vi "Bloomy BS120x Configuration Example.vi"() -> ()   [LabVIEW 2021]
uses:
  src/TypeDefs/UnitType.ctl
  src/TypeDefs/CAN Settings.ctl
  src/TypeDefs/Ethernet Settings.ctl
  src/TypeDefs/Protocol.ctl
  src/Public/New BS120x Device/New BS120x Ethernet Device.vi
  src/BS120x.lvclass
  src/BS120x Driver.lvlib
panel:
  out "reset status":string
  out "Cell Inhibit Enable":bool
  in  "Cell Inhibit Enable":bool
  out "error out":errorcluster
  in  "Reset Unit":bool
  in  "Update IP":bool
  in  "New IP Address":string="192.168.1.100"
  in  "Update Config":bool
  in  "New Protocol (Legacy)":T1 caption="Protocol (Legacy)"
  in  "New Ethernet Settings":T2 caption="Ethernet Settings"
  in  "New CAN Settings":T3 caption="CAN Settings"
  out "Calibration Date":string
  out "SerialNumber":string
  out "Firmware":string
  out "Protocol (Legacy)":T1
  out "Ethernet Settings":T2
  out "CAN Settings":T3
  in  "Retrieve Config":bool
  in  "Box IP address":string="192.168.1.101"
  in  "TCP port":u16=12345
  in  "UDP port":u16=54321
  in  "Unit Type":T4=enum."BS1201"
  in  "stop":bool
  # "Initialization & Configuration"
  # "New Configuration"
  # "Ethernet Only"
  # "Changes do not take effect until unit is reset"
  # "Current Configuration"
  # "Automatically resets unit"
  # "(c) 2024 Bloomy Controls, Inc. All rights reserved."
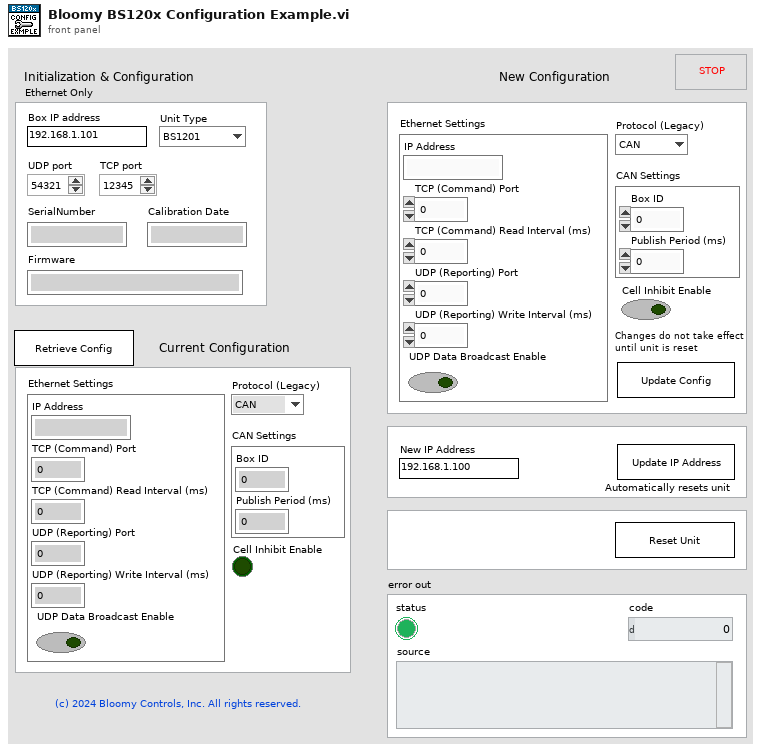
[diagram p1: front panel]
types:
  T1 = typedef "BS120x Driver.lvlib/BS120x.lvclass/Protocol.ctl" = enum16{"CAN", "Ethernet"}
  T2 = typedef "BS120x Driver.lvlib/BS120x.lvclass/Ethernet Settings.ctl" = cluster{"IP Address":string, "TCP (Command) Port":u16, "TCP (Command) Read Interval (ms)":u32, "UDP (Reporting) Port":u16, "UDP (Reporting) Write Interval (ms)":u32, "UDP Data Broadcast Enable":bool}
  T3 = typedef "BS120x Driver.lvlib/BS120x.lvclass/CAN Settings.ctl" = cluster{"Box ID":i32, "Publish Period (ms)":i32}
  T4 = typedef "BS120x Driver.lvlib/BS120x.lvclass/UnitType.ctl" = enum16{"BS1200", "BS1201"}
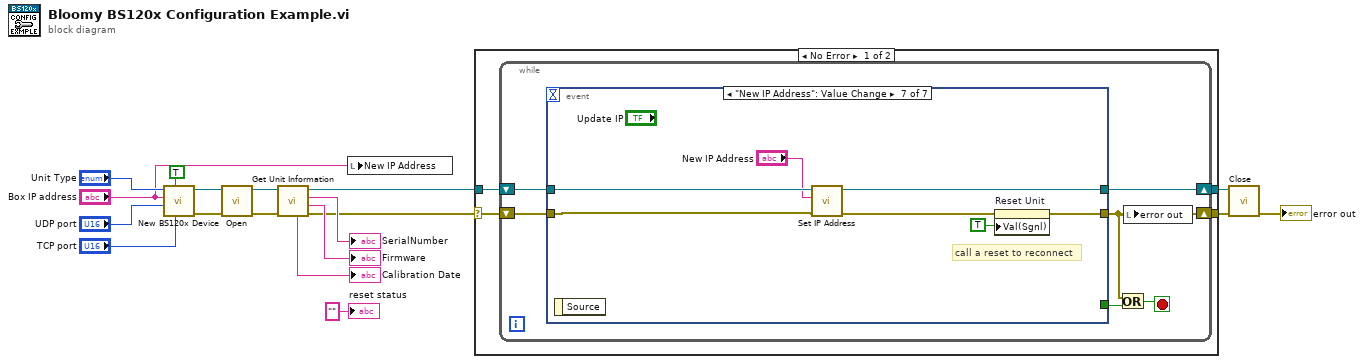
[diagram p0: block diagram]
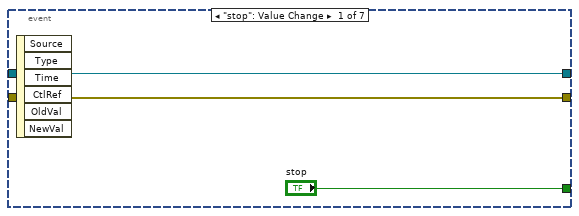
[diagram p2: hidden frame]
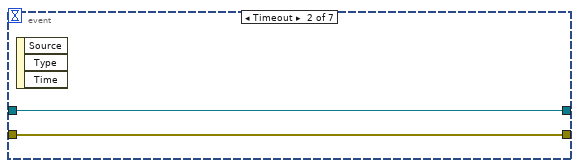
[diagram p3: hidden frame]
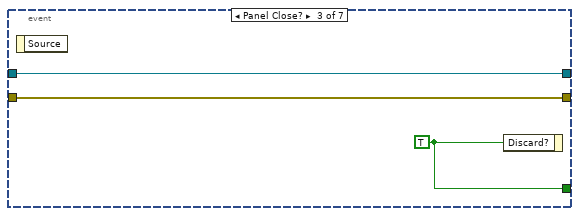
[diagram p4: hidden frame]
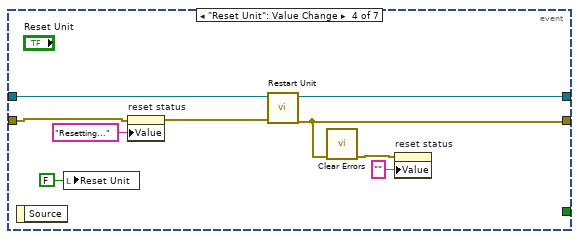
[diagram p5: hidden frame]
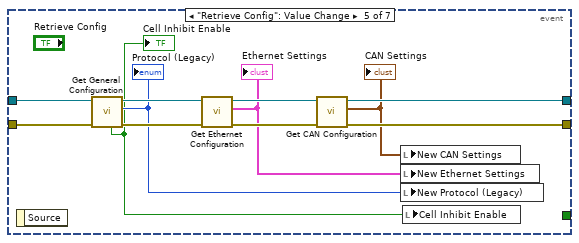
[diagram p6: hidden frame]
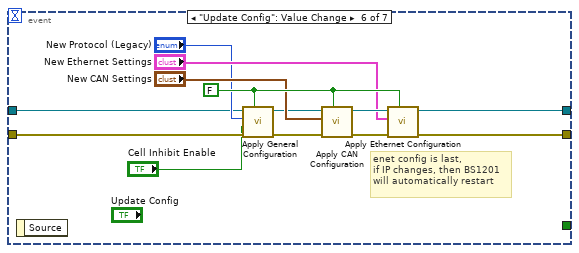
[diagram p7: hidden frame]
diagram:
  n1 = call-poly "New BS120x Device.vi"("TCP port"="TCP port", "Connect for Config Only? (F)"=TRUE, "UDP port"="UDP port", "Box IP address"="Box IP address", "Unit Type"="Unit Type") -> ("error out"=w8:errorcluster, "BS120x Out"=w9:refnum<class "BS120x.lvclass">)  [unwired: 5 in]
  n2 = call-dynamic "Open.vi"("error in (no error)"=w8, "BS120x in"=w9) -> ("error out"=w7:errorcluster, "BS120x out"=w6:refnum<class "BS120x.lvclass">)  [unwired: 8 in]
  n3 = call-dynamic "Get Unit Information.vi"("error in (no error)"=w7, "BS120x in"=w6) -> ("error out"=w2:errorcluster, "Firmware"=→"Firmware":string, "SerialNumber"=→"SerialNumber":string, "BS120x out"=w13:refnum<class "BS120x.lvclass">, "Calibration Date"=→"Calibration Date":string)  [unwired: 5 in]
  n4 = local write "New IP Address"("Box IP address") -> ()
  n5 = case shown="No Error" w2 {
    selector: w2 -> [w19 w78]
    tunnel: [w22 w78] -> w18
    tunnel: [w21 w79] -> w17
    tunnel: w13 -> [w20 w79]
    frame No Error {
      n6 = while {
        shift-right: [w23] -> w22
        shift-left: w19 -> [w26]
        shift-right: [w28] -> w21
        shift-left: w20 -> [w27]
        stop <- w25 stop-if-true
        n7 = event shown="[6] \"New IP Address\": Value Change" {
          selector: _ -> [_ _ _ _ _ _ _]
          dyn-events: _ -> [_ _ _ _ _ _ _]
          timeout: _ -> [_ _ _ _ _ _ _]
          tunnel: [w31 w33 w36 w45 w51 w64 w76] -> w28
          tunnel: w27 -> [w31 w33 w36 w44 w57 w60 w77]
          tunnel: [w30 w32 w34 w40 w50 w63 w72] -> w23
          tunnel: w26 -> [w30 w32 w34 w42 w56 w59 w74]
          tunnel: ["stop" _ w35 _ _ _ _] -> w24
          event "stop": Value Change {
            n8 = event-data() -> ()  [unwired: 1 in, 6 out]
          }
          event Timeout {
            n9 = event-data() -> ()  [unwired: 1 in, 3 out]
          }
          event Panel Close? {
            w35 = TRUE ("Discard?")
            n10 = event-data() -> ()  [unwired: 1 in, 1 out]
            n11 = event-data("Discard?"=w35) -> ()  [unwired: 1 in, 1 out]
          }
          event "Reset Unit": Value Change {
            n12 = event-data() -> ()  [unwired: 1 in, 1 out]
            n13 = local write "Reset Unit"(FALSE ("Reset Unit")) -> ()
            n14 = property on="reset status" class="Str"(error in=w42, "Value"="Resetting..." ("reset status")) -> (error out=w41:errorcluster)  [unwired: 1 in, 1 out]
            n15 = call-dynamic "Restart Unit.vi"("error in (no error)"=w41, "BS120x in"=w44) -> ("error out"=w40:errorcluster, "BS120x out"=w45:refnum<class "BS120x.lvclass">)  [unwired: 8 in]
            n16 = call <vilib>:"Clear Errors.vi"("error in (no error)"=w40) -> ("error out"=w38:errorcluster)  [unwired: 5 in, 1 out]
            n17 = property on="reset status" class="Str"(error in=w38, "Value"="" ("reset status")) -> ()  [unwired: 1 in, 2 out]
          }
          event "Retrieve Config": Value Change {
            n18 = event-data() -> ()  [unwired: 1 in, 1 out]
            n19 = call-dynamic "Get General Configuration.vi"("error in (no error)"=w56, "BS120x in"=w57) -> ("error out"=w54:errorcluster, "Protocol"=w47:T1, "BS120x out"=w55:refnum<class "BS120x.lvclass">, "Cell Inhibit Enable"=w46:bool)  [unwired: 5 in, 1 out]
            "Protocol (Legacy)" <- w47
            "Cell Inhibit Enable" <- w46
            n20 = call-dynamic "Get Ethernet Configuration.vi"("error in (no error)"=w54, "BS120x in"=w55) -> ("error out"=w52:errorcluster, "Ethernet Settings"=w48:T2, "BS120x out"=w53:refnum<class "BS120x.lvclass">)  [unwired: 6 in, 1 out]
            "Ethernet Settings" <- w48
            n21 = call-dynamic "Get CAN Configuration.vi"("error in (no error)"=w52, "BS120x in"=w53) -> ("error out"=w50:errorcluster, "CAN Settings"=w49:T3, "BS120x out"=w51:refnum<class "BS120x.lvclass">)  [unwired: 6 in, 1 out]
            "CAN Settings" <- w49
            n22 = local write "New CAN Settings"(w49) -> ()
            n23 = local write "New Ethernet Settings"(w48) -> ()
            n24 = local write "New Protocol (Legacy)"(w47) -> ()
            n25 = local write "Cell Inhibit Enable"(w46) -> ()
          }
          event "Update Config": Value Change {
            w68 = FALSE ("Restart (T)")
            # "enet config is last,\nif IP changes, then BS1201\nwill automatically restart"
            n26 = event-data() -> ()  [unwired: 1 in, 1 out]
            n27 = call-dynamic "Apply General Configuration.vi"("Restart (T)"=w68, "error in (no error)"=w59, "Cell Inhibit Enable"="Cell Inhibit Enable", "Protocol (Legacy)"="New Protocol (Legacy)", "BS120x in"=w60) -> ("error out"=w61:errorcluster, "BS120x out"=w62:refnum<class "BS120x.lvclass">)  [unwired: 5 in]
            n28 = call-dynamic "Apply CAN Configuration.vi"("Restart (T)"=w68, "error in (no error)"=w61, "CAN Settings"="New CAN Settings", "BS120x in"=w62) -> ("error out"=w69:errorcluster, "BS120x out"=w70:refnum<class "BS120x.lvclass">)  [unwired: 6 in]
            n29 = call-dynamic "Apply Ethernet Configuration.vi"("Restart (T)"=w68, "error in (no error)"=w69, "Ethernet Settings"="New Ethernet Settings", "BS120x in"=w70) -> ("error out"=w63:errorcluster, "BS120x out"=w64:refnum<class "BS120x.lvclass">)  [unwired: 6 in]
          }
          event "New IP Address": Value Change {
            # "call a reset to reconnect"
            n30 = event-data() -> ()  [unwired: 1 in, 1 out]
            n31 = call-dynamic "Set IP Address.vi"("error in (no error)"=w74, "IP Address"="New IP Address", "BS120x in"=w77) -> ("error out"=w73:errorcluster, "BS120x out"=w76:refnum<class "BS120x.lvclass">)  [unwired: 7 in]
            n32 = property on="Reset Unit" class="Bool (strict)"(error in=w73, "Val(Sgnl)"=TRUE ("Value (Signaling)")) -> (error out=w72:errorcluster)  [unwired: 1 in, 1 out]
          }
        }
        n33 = Or(x=w23, y=w24) -> (x .or. y?=w25:bool)
        n34 = local write "error out"(w23) -> ()
      }
    }
    frame Error {
    }
  }
  n35 = call-dynamic "Close.vi"("error in (no error)"=w18, "BS120x In"=w17) -> ("error out"=→"error out":errorcluster)  [unwired: 8 in, 1 out]
  "reset status" <- "" ("reset status")
